vi "Coral Get Next State.vi"(11 "Coral Main Cluster in":T2={"Coral FIFO"=[], "Camera Name"="", "Coral path"=path "", "Control Ref's"=[], "Greyscale Mask Image"=refnum, "Main Image"=refnum, "Coral Color Range"={"Hue"={21.620689392089844, 69.62068939208984}, "Sat"={66.41378784179688, 255.0}, "Val"={96.0, 255.0}}, "Timeout"=5} {"Coral Color Range"."Hue" scale=0.0..255.0 scale format="%#_3g"}) -> (1 "Next State":T1, 3 "Coral Main Cluster out":T2={"Coral FIFO"=[], "Camera Name"="", "Coral path"=path "", "Control Ref's"=[], "Greyscale Mask Image"=refnum, "Main Image"=refnum, "Coral Color Range"={"Hue"={21.620689392089844, 69.62068939208984}, "Sat"={66.41378784179688, 255.0}, "Val"={96.0, 255.0}}, "Timeout"=5} {"Coral Color Range"."Hue" scale=0.0..255.0 scale format="%#_3g"})   [LabVIEW 2025]
uses:
  Coral Main CLuster.ctl
  Coral States.ctl
  <vilib>/vision/Image Controls.llb/IMAQ Image.ctl
  Ball/State Machine/Ball States.ctl
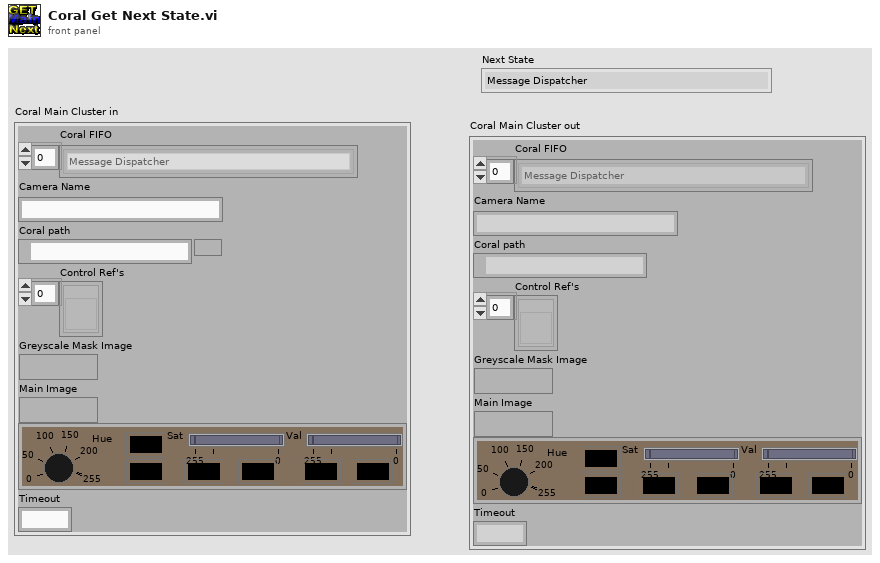
[diagram p1: front panel]
types:
  T1 = typedef "Ball States.ctl" = enum16{"Message Dispatcher", "INI", "Open", "Save", "Exit"}
  T2 = typedef "Coral Main CLuster.ctl" = cluster{"Coral FIFO":T3[], "Camera Name":string, "Coral path":path, "Control Ref's":refnum<vi>[], "Greyscale Mask Image":T4, "Main Image":T4, "Coral Color Range":cluster{"Hue":cluster{dbl, dbl}, "Sat":cluster{dbl, dbl}, "Val":cluster{dbl, dbl}}, "Timeout":i32}
  T3 = typedef "Coral States.ctl" = enum16{"Message Dispatcher", "INI", "Open", "Save", "Exit"}
  T4 = typedef "IMAQ Image.ctl" = refnum<image>
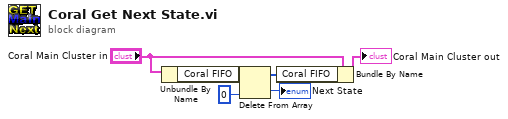
[diagram p0: block diagram]
diagram:
  n1 = Unbundle By Name("Coral Main Cluster in") -> ("Coral FIFO"=w6:T3[])
  n2 = Delete From Array(array=w6, index=0) -> (deleted portion=→"Next State":T3, array with subset deleted=w3:T3[])  [unwired: 1 in]
  n3 = Bundle By Name(cluster="Coral Main Cluster in", "Coral FIFO"=w3) -> (→"Coral Main Cluster out":T2)
